vi "Rotate.vi"(8 "error in (no error)":errorcluster, 10 "angle":sgl, 11 "Canvas in":refnum<class "Drawer .Net.lvclass">) -> (0 "error out":errorcluster, 3 "Canvas out":refnum<class "Drawer .Net.lvclass">)   [LabVIEW 2023, in "Glyph .NET Drawer.lvlib" / "Drawer .Net.lvclass"]
uses:
  Drawer .Net.lvclass
  Drawer .Net.lvclass/Drawer .Net.ctl
  System.Drawing
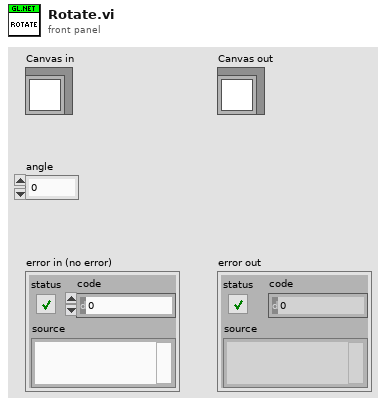
[diagram p1: front panel]
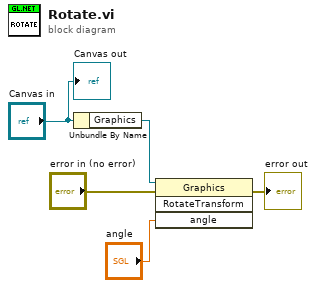
[diagram p0: block diagram]
diagram:
  n1 = Unbundle By Name("Canvas in") -> ("Graphics"=w1:refnum<k24>)
  n2 = invoke class="Graphics" method="RotateTransform"(reference=w1, error in="error in (no error)", "angle"="angle") -> (error out=→"error out":errorcluster)  [unwired: 1 in, 3 out]
  "Canvas out" <- "Canvas in"
